vi "Palindrome_ID.vi"() -> ()   [LabVIEW 2022 SP3]
panel:
  out "Palindrome?":bool
  in  "Enter a word:":string
  # "Palindrome_ID\nEnter a word in the field below,\nif that word is a palindrome, the \nLED will turn green."
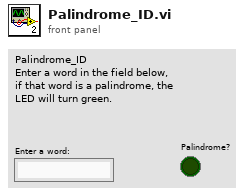
[diagram p1: front panel]
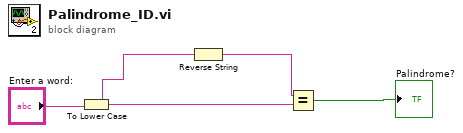
[diagram p0: block diagram]
diagram:
  n1 = To Lower Case(string="Enter a word:") -> (all lower case string=w2:string)
  n2 = Reverse String(1:w2) -> (0:w3:string)
  n3 = Equal?(x=w3, y=w2) -> (x = y?=→"Palindrome?":bool)
